vi "read_position.vi"(8 "error in (no error)":errorcluster, 11 "VISA resource name":refnum<visa-resource-name>) -> (0 "error out":errorcluster, 2 "position (s)":dbl, 3 "VISA resource name out":refnum<visa-resource-name>)   [LabVIEW 2017, in "lecroy.lvlib"]
doc: "Read the attenuation factor of the specified channel."
uses:
  lecroy.lvlib
  <instrlib>/LeCroy Wave Series/LeCroy Wave Series.lvlib
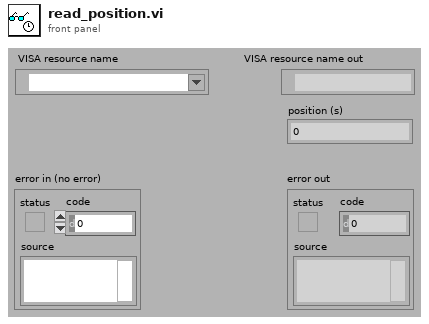
[diagram p1: front panel]
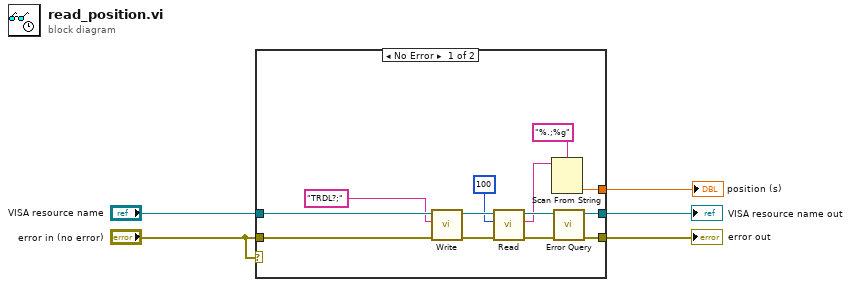
[diagram p0: block diagram]
diagram:
  n1 = case shown="No Error" "error in (no error)" {
    tunnel: "VISA resource name" -> [w15 w20]
    tunnel: "error in (no error)" -> [w14 w19]
    tunnel: [w11 w20] -> w4
    tunnel: [w10 w19] -> w3
    tunnel: [w7 _] -> w2
    frame No Error {
      n2 = call <instrlib>:"Write.vi"("error in (no error)"=w14, "Write Buffer"="TRDL?;", "VISA resource name"=w15) -> ("error out"=w18:errorcluster, "VISA resource name out"=w17:refnum<visa-resource-name>)  [unwired: 6 in, 1 out]
      n3 = call <instrlib>:"Read.vi"("error in (no error)"=w18, "Byte Count"=u32 100, "VISA resource name"=w17) -> ("error out"=w12:errorcluster, "Read Buffer"=w8:string, "VISA resource name out"=w13:refnum<visa-resource-name>)  [unwired: 5 in, 1 out]
      n4 = Scan From String(format string="%.;%g", input string=w8) -> (output 1=w7:dbl)  [unwired: 3 in, 3 out]
      n5 = call <instrlib>:"Error Query.vi"("error in (no error)"=w12, "VISA resource name"=w13) -> ("error out"=w10:errorcluster, "VISA resource name out"=w11:refnum<visa-resource-name>)  [unwired: 6 in, 2 out]
    }
    frame Error {
    }
  }
  "error out" <- w3
  "VISA resource name out" <- w4
  "position (s)" <- w2
